vi "Display Image.vi"(8 "error in (no error)":errorcluster, 9 "Image Indicator":refnum<vi>, 10 "File Name":string, 11 "Controller in":refnum<class "Controller.lvclass">) -> (0 "error out":errorcluster, 3 "Controller out":refnum<class "Controller.lvclass">)   [LabVIEW 2022 SP3, in "Controller.lvlib" / "Controller.lvclass"]
uses:
  Controller.lvclass
  Controller.lvclass/Controller.ctl
  ImageHandler/ImageHandler Messages/Display Image Msg/Display Image Msg.lvclass/Display Image Msg.ctl
  <vilib>/ActorFramework/Message Enqueuer/Message Enqueuer.lvclass/Message Enqueuer.ctl
  <vilib>/ActorFramework/Message Enqueuer/Enqueue.vi
  ImageHandler/ImageHandler Messages/Display Image Msg/Display Image Msg.lvclass
  C:/Program Files/National Instruments/LabVIEW 2022/vi.lib/ActorFramework/Message/Message.lvclass
  <vilib>/ActorFramework/Message Priority Queue/Priority Enqueue.vi
  <vilib>/ActorFramework/Message Enqueuer/Message Enqueuer.lvclass
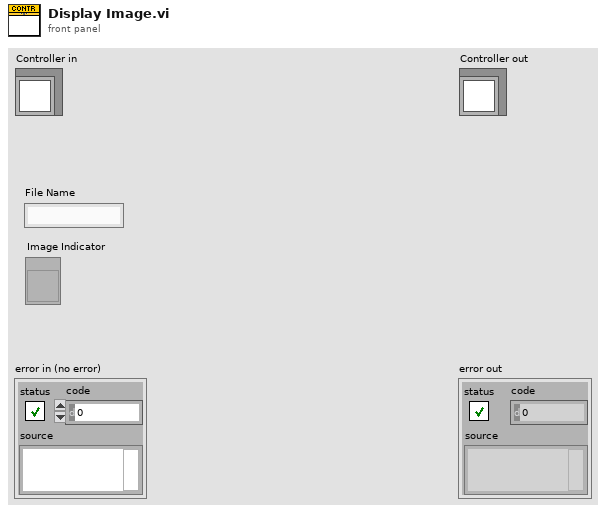
[diagram p1: front panel]
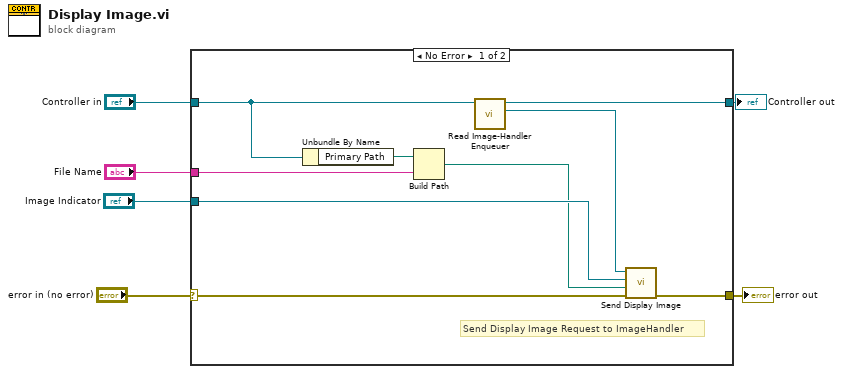
[diagram p0: block diagram]
diagram:
  n1 = case shown="No Error" "error in (no error)" {
    selector: "error in (no error)" -> [w10 w16]
    tunnel: [w9 w16] -> w5
    tunnel: "Controller in" -> [w15 w17]
    tunnel: [w8 w17] -> w3
    tunnel: "File Name" -> [w13 _]
    tunnel: "Image Indicator" -> [w12 _]
    frame No Error {
      # "Send Display Image Request to ImageHandler"
      n2 = Unbundle By Name(w15) -> ("Primary Path"=w14:path)
      n3 = Build Path(base path=w14, name or relative path=w13) -> (appended path=w11:path)
      n4 = call "Read Image-Handler Enqueuer.vi"("Controller in"=w15) -> ("Actor Framework:Message Enqueuer"=w7:refnum<class "Message Enqueuer.lvclass">, "Controller out"=w8:refnum<class "Controller.lvclass">)  [unwired: 8 in, 1 out]
      n5 = call "Send Display Image.vi"("error in (no error)"=w10, "Path"=w11, "Image Indicator"=w12, "Message Enqueuer"=w7) -> ("error out"=w9:errorcluster)  [unwired: 6 in, 1 out]
    }
    frame Error {
    }
  }
  "error out" <- w5
  "Controller out" <- w3
